vi "TestSCAN.vi"(8 "errin":errorcluster) -> (0 "error out":errorcluster, 2 "COM VUS":refnum<visa-resource-name>[](array[refnum]), 3 "Retour IDN":string[](array[string]))   [LabVIEW 2020]
doc: "Ce VI te sniff tout les équipement VISA qu'il détect et t'en fait une liste"
uses:
  <vilib>/Instr/_visa.llb/VISA Find Search Mode.ctl
  <vilib>/MakerHub/LINX/Public/Utilities/Open Serial.vi
  <vilib>/MakerHub/LINX/LMH-LINX.lvlib
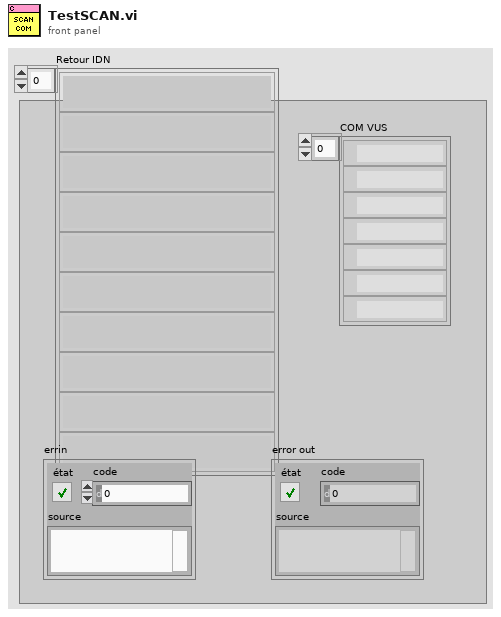
[diagram p1: front panel]
types:
  T1 = typedef "VISA Find Search Mode.ctl" = u32
  T2 = typedef "LMH-LINX.lvlib/LINX Ref.ctl" = cluster{"IO":T3, "Interface":T4, "LINX Device Config":T5}
  T3 = typedef "LMH-LINX.lvlib/Platform.ctl" = enum16{"Remote", "Local"}
  T4 = typedef "LMH-LINX.lvlib/Interface.ctl" = enum16{"Serial", "TCP"}
  T5 = typedef "LMH-LINX.lvlib/Device.lvlib/LINX Device Config.ctl" = cluster{"Interface":T4, "COM Port":refnum<visa-resource-name>, "TCP Configuration":T6, "Device Family":u8, "Device ID":u8, "Device Name":string, "TCP Ref":refnum<k5>, "Channels":T7}
  T6 = typedef "LMH-LINX.lvlib/Device.lvlib/TCP Config.ctl" = cluster{"IP Address":string, "Port":u16}
  T7 = typedef "LMH-LINX.lvlib/Channels.ctl" = cluster{"DI":u8[], "DO":u8[], "AI":u8[], "AO":u8[], "PWM":u8[], "QE":u8[], "UART":u8[], "I2C 2":u8[], "SPI":u8[], "CAN":u8[], "Servo":u8[], "AI Ref (V)":dbl, "AI Resolution (Bits)":u8, "AO Ref (V)":dbl, "AO Resolution (Bits)":u8}
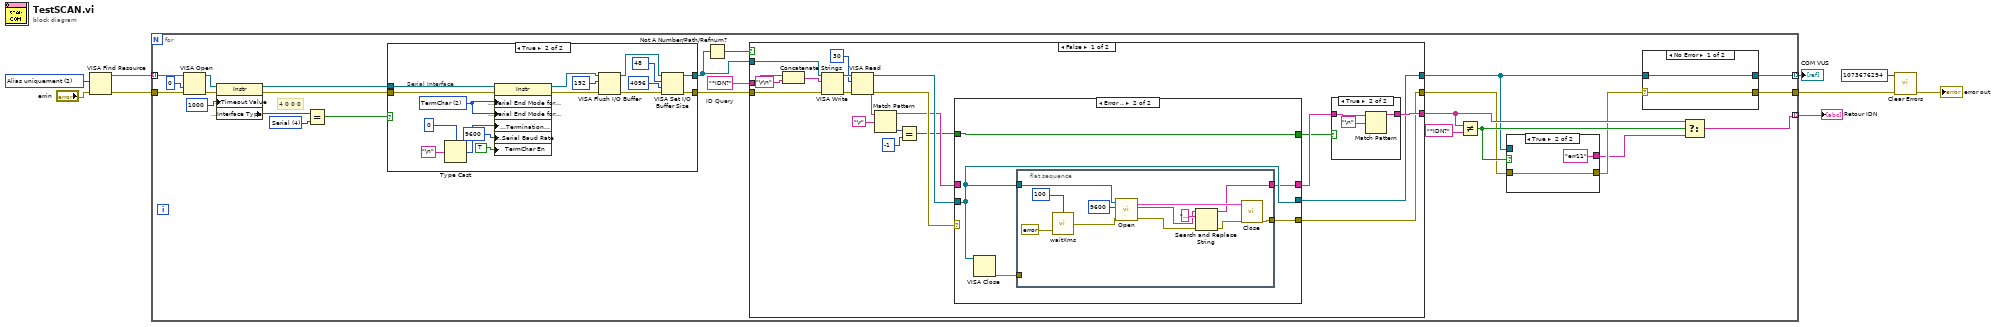
[diagram p0: block diagram]
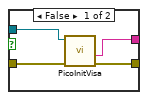
[diagram p2: hidden frame]
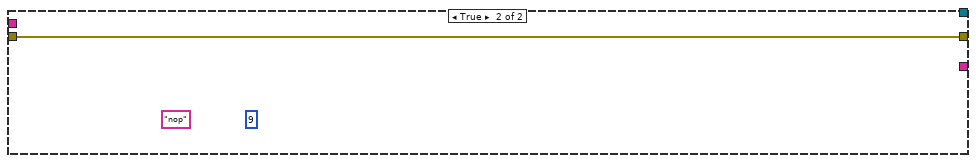
[diagram p5: hidden frame]
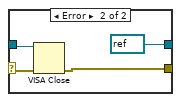
[diagram p7: hidden frame]
diagram:
  w5 = T1 2 items=["Noms canoniques uniquement"=0, "Alias uniquement"=2, "Inclure les alias correspondants"=3, "Inclure tous les alias"=4] ("Search Mode")
  n1 = VISA Find Resource(8:"errin", 10:w5) -> (0:w4:errorcluster, 3:w9:string[])  [unwired: 1 in, 1 out]
  n2 = for {
    tunnel: w9 -> [w27] mode=indexing
    tunnel: [w13] -> w8 mode=indexing
    tunnel: [w22] -> w6 mode=indexing
    tunnel: w4 -> [w26]
    tunnel: [w23] -> w3
    w24 = "*IDN?"  # ID Query
    w21 = u16 4 items=["GPIB"=1, "VXI"=2, "GPIB-VXI"=3, "Serial"=4, "PXI"=5, "TCPIP"=6, "USB"=7] ("Interface Information:Interface Type")
    # "4 0 0 0"
    n3 = VISA Open(access mode=u32 0, error in (no error)=w26, VISA resource name=w27) -> (VISA resource name=w29:refnum<visa-resource-name>, error out=w28:errorcluster)  [unwired: 2 in]
    n4 = property class="Instr"(reference=w29, error in=w28, "General Settings:Timeout Value"=u32 1000) -> (reference out=w32:refnum<visa-resource-name>, error out=w31:errorcluster, "Interface Information:Interface Type"=w12:u16)
    n5 = Equal?(x=w12, y=w21) -> (x = y?=w10:bool)
    n6 = case shown="True" w10 {
      tunnel: [w88 w103] -> w33
      tunnel: [w89 w100] -> w11
      tunnel: w32 -> [w88 w105]
      tunnel: w31 -> [w89 w106]
      frame False {
        # "EDIT: Remove interfaces not supported by your instrument."
        # "GPIB, TCP/IP, and USB Interface"
      }
      frame True {
        w93 = u16 2 items=["None", "LastBit", "TermChar"] ("Serial Settings:Serial End Mode for Reads")
        # "Serial Interface"
        n7 = Type Cast(type=u8 0, x="\n" ("Line Feed Constant")) -> (*(type *) &x=w92:u8)
        n8 = property class="Instr"(reference=w105, error in=w106, "Serial Settings:Serial End Mode for Reads"=w93, "Serial Settings:Serial End Mode for Writes"=w93, "Message Based Settings:Termination Character"=w92, "Serial Settings:Serial Baud Rate"=u32 9600 ("Serial Settings:Baud Rate"), "TermChar En"=TRUE ("Message Based Settings:Termination Character Enable")) -> (reference out=w99:refnum<visa-resource-name>, error out=w102:errorcluster)
        n9 = VISA Flush I/O Buffer(VISA resource name=w99, mask (16)=u16 192, error in (no error)=w102) -> (VISA resource name out=w104:refnum<visa-resource-name>, error out=w101:errorcluster)
        n10 = VISA Set I/O Buffer Size(VISA resource name=w104, mask (16)=u16 48, size (4096)=u32 4096 ("size (0)"), error in (no error)=w101) -> (VISA resource name out=w103:refnum<visa-resource-name>, error out=w100:errorcluster)
      }
    }
    n11 = Not A Number/Path/Refnum?(number/path/refnum=w33) -> (NaN/Path/Refnum?=w25:bool)
    n12 = case shown="False" w25 {
      tunnel: [w45 _] -> w15
      tunnel: [w47 w87] -> w17
      tunnel: [w55 _] -> w19
      tunnel: w33 -> [w48 _]
      tunnel: w24 -> [w54 _]
      tunnel: w11 -> [w52 w87]
      frame False {
        n13 = Concatenate Strings(w54, "\r\n") -> (w58:string)
        n14 = VISA Write(VISA resource name=w48, write buffer=w58, error in (no error)=w52) -> (VISA resource name out=w61:refnum<visa-resource-name>, error out=w60:errorcluster)  [unwired: 1 out]
        n15 = VISA Read(VISA resource name=w61, byte count=u32 30 ("nombre d'octets"), error in (no error)=w60) -> (VISA resource name out=w46:refnum<visa-resource-name>, read buffer=w51:string, error out=w49:errorcluster)  [unwired: 1 out]
        n16 = Match Pattern(string=w51, regular expression="\r") -> (before substring=w44:string, offset past match=w50:i32)  [unwired: 1 in, 2 out]
        n17 = Equal?(x=w50, y=-1) -> (x = y?=w42:bool)
        n18 = case shown="Error .." w49 {
          selector: w49 -> [w65 _]
          tunnel: w46 -> [w64 w68]
          tunnel: [w65 w70] -> w47
          tunnel: [w64 w68] -> w45
          tunnel: w44 -> [w63 _]
          tunnel: [w63 w66] -> w43
          tunnel: w42 -> [w62 w67]
          tunnel: [w62 w67] -> w41
          frame No Error {
          }
          frame Error {
            n19 = VISA Close(VISA resource name=w68) -> (error out=w69:errorcluster)  [unwired: 1 in]
            n20 = flat-sequence {
              tunnel: [w81] -> w70
              tunnel: w69 -> [_]
              tunnel: w68 -> [w76]
              tunnel: [w73] -> w66
              frame #0 {
                n21 = call <userlib>:"waitXms.vi"("attente (ms)"=u32 100, "errin"=errorcluster {"status"=FALSE, "code"=0, "source"=""} ("Error In")) -> ("errout"=w78:errorcluster)  [unwired: 13 in]
                n22 = call-poly <vilib>:"Open.vi"("Error In"=w78, "Baud Rate Override"=u32 9600, "Serial Port"=w76) -> ("Error Out"=w72:errorcluster, "Device Name"=w74:string, "LINX Resource"=w82:T2)  [unwired: 6 in]
                n23 = Search and Replace String ("Rechercher et remplacer une chaîne")(input string=w74, search string="\u0000" ("chaîne recherchée"), error in=w72) -> (result string=w73:string, error out=w71:errorcluster)  [unwired: 5 in, 2 out]
                n24 = call <vilib>:"Close.vi"("Error In"=w71, "LINX Resource"=w82) -> ("Error Out"=w81:errorcluster)  [unwired: 9 in]
              }
            }
          }
        }
        n25 = case shown="True" w41 {
          tunnel: w43 -> [w83 w85]
          tunnel: [w83 w84] -> w55
          frame False {
          }
          frame True {
            n26 = Match Pattern(string=w85, regular expression="\n") -> (before substring=w84:string)  [unwired: 1 in, 3 out]
          }
        }
      }
      frame True {
        (unwired) 9 ("offset past match")
        (unwired) "nop" ("read buffer")
      }
    }
    n27 = Not Equal?(x=w19, y="*IDN?") -> (x != y?=w18:bool)
    n28 = case shown="True" w18 {
      tunnel: w17 -> [w38 w40]
      tunnel: [w37 w40] -> w16
      tunnel: w15 -> [w36 _]
      tunnel: [w35 "err11" ("data out")] -> w14
      frame False {
        n29 = call "PicoInitVisa.vi"("errin"=w38, "visain"=w36) -> ("sortie d'erreur"=w37:errorcluster, "buffer de lecture 2"=w35:string)  [unwired: 6 in, 2 out]
      }
      frame True {
      }
    }
    n30 = case shown="No Error" w16 {
      selector: w16 -> [w107 w111]
      tunnel: w15 -> [w108 w110]
      tunnel: [w108 refnum<visa-resource-name> refnum ("VISA resource name out")] -> w22
      tunnel: [w107 w109] -> w23
      frame No Error {
      }
      frame Error {
        n31 = VISA Close(VISA resource name=w110, error in (no error)=w111) -> (error out=w109:errorcluster)
      }
    }
    n32 = Select(t=w19, s=w18, f=w14) -> (s? t:f=w13:string)
  }
  "Retour IDN" <- w8
  "COM VUS" <- w6
  n33 = call <vilib>:"Clear Errors.vi"("error in (no error)"=w3, "specific error code to clear (0: all)"=1073676294) -> ("error out"=→"error out":errorcluster)  [unwired: 4 in, 1 out]
